vi "SET_Layer_Data.vi"(6 "Layer Tab Value Change? (F)":bool, 8 "error in (no error)":errorcluster, 10 "Data":T1={"LayerIcon"=bytes[3102], "LayerName"="", "Opacity"=100, "Visibility?"=TRUE} {"Opacity" scale=0.0..100.0}, 11 "Layer.lvclass in":refnum<class "Layer.lvclass">) -> (0 "error out":errorcluster, 3 "Layer.lvclass out":refnum<class "Layer.lvclass">)   [LabVIEW 2020, in "Layer.lvclass"]
doc: "Sets the User Layer data. This VI preserves the data for Origina and Type."
uses:
  <vilib>/LabVIEW Icon API/lv_icon/Classes/Layer/Layer.lvclass
  <vilib>/LabVIEW Icon API/lv_icon/Controls/Layer.ctl
  <vilib>/LabVIEW Icon API/lv_icon/Classes/Layer/Layer.lvclass/Layer.ctl
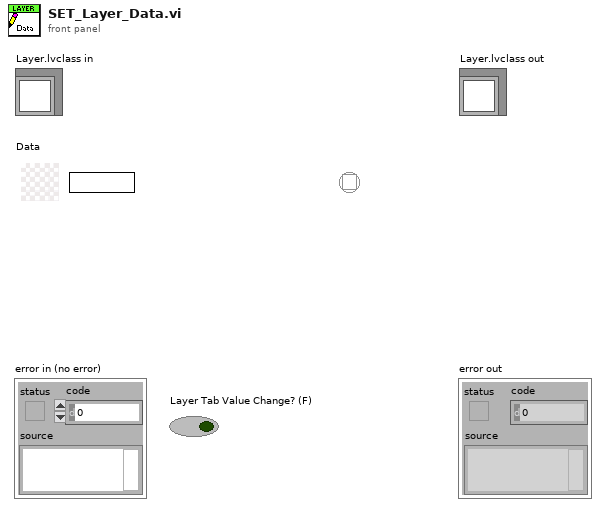
[diagram p1: front panel]
types:
  T1 = typedef "Layer.ctl" = cluster{"LayerIcon":picture, "LayerName":string, "Opacity":u8, "Visibility?":bool}
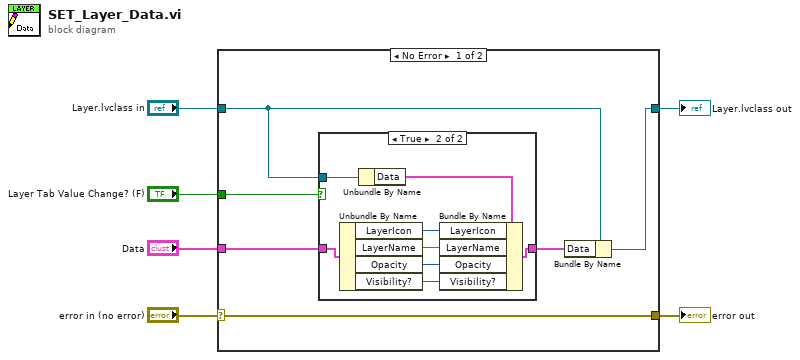
[diagram p0: block diagram]
diagram:
  n1 = case shown="No Error" "error in (no error)" {
    selector: "error in (no error)" -> [w12 w22]
    tunnel: [w12 w22] -> w5
    tunnel: [w11 w23] -> w3
    tunnel: "Layer.lvclass in" -> [w9 w23]
    tunnel: "Data" -> [w8 _]
    tunnel: "Layer Tab Value Change? (F)" -> [w10 _]
    frame No Error {
      n2 = case shown="True" w10 {
        tunnel: w9 -> [_ w21]
        tunnel: w8 -> [w13 w20]
        tunnel: [w13 w15] -> w7
        frame False {
        }
        frame True {
          n3 = Unbundle By Name(w20) -> ("LayerIcon"=w18:picture, "LayerName"=w17:string, "Opacity"=w16:u8, "Visibility?"=w14:bool)
          n4 = Unbundle By Name(w21) -> ("Data"=w19:T1)
          n5 = Bundle By Name(cluster=w19, "LayerIcon"=w18, "LayerName"=w17, "Opacity"=w16, "Visibility?"=w14) -> (w15:T1)
        }
      }
      n6 = Bundle By Name(cluster=w9, "Data"=w7) -> (w11:refnum<class "Layer.lvclass">)
    }
    frame Error {
    }
  }
  "error out" <- w5
  "Layer.lvclass out" <- w3
